vi "Turbo Boost.vi"(4 "Normal Speed Constant":dbl, 5 "Turbo Activate Button":bool, 6 "Y Axis Joystick Input":dbl, 7 "X Axis Joystick Input":dbl) -> (2 "Y Axis New Value":dbl, 3 "X Axis New Value":dbl)   [LabVIEW 2019]
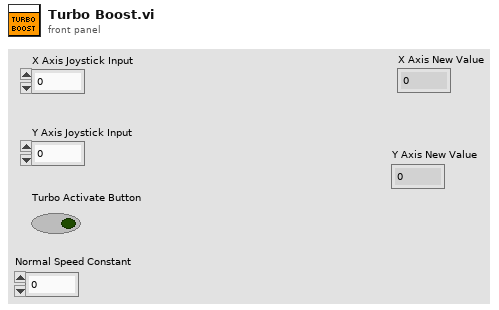
[diagram p1: front panel]
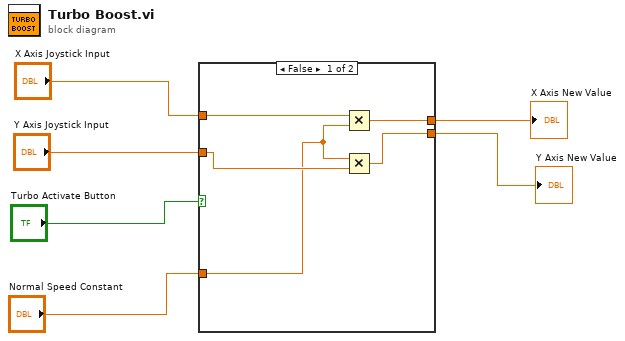
[diagram p0: block diagram]
diagram:
  n1 = case shown="False" "Turbo Activate Button" {
    tunnel: "X Axis Joystick Input" -> [w9 w13]
    tunnel: "Y Axis Joystick Input" -> [w8 w12]
    tunnel: "Normal Speed Constant" -> [w7 _]
    tunnel: [w11 w13] -> w1
    tunnel: [w10 w12] -> w2
    frame False {
      n2 = Multiply(x=w9, y=w7) -> (x*y=w11:dbl)
      n3 = Multiply(x=w7, y=w8) -> (x*y=w10:dbl)
    }
    frame True {
    }
  }
  "X Axis New Value" <- w1
  "Y Axis New Value" <- w2
